vi "PID+calculation.vi"() -> ()   [LabVIEW 2020]
uses:
  Control 1.ctl
  <vilib>/Instr/_visa.llb/VISA Configure Serial Port (Instr).vi
panel:
  in  "Accept":bool
  out "Autotuned":T1
  out "T":dbl=50.98039215686275
  out "L":dbl
  out "Autotune\narray":dbl[](array[numeric])
  in  "Autotune":bool
  out "dt":dbl
  out "String":string
  out "error":dbl=19.0
  out "Error":bool
  out "Numeric":i32=4582
  out "result":dbl(knob)=1.1028626441956932 scale=0.0..255.0
  out "lasterror":dbl=0.010000000000001563
  out "cumError":dbl=0.001016087532043616
  out "previous time":timestamp=timestamp(3700781718.785231 s since 1904-01-01)
  in  "PID Gains":T1={"Proportional Gain(Kp)"=80.0, "Integral Gain(Ki)"=100.0, "Differential Gain(Kd)"=0.0} {"Differential Gain(Kd)" format="%#.6g"; "Integral Gain(Ki)" format="%#.6g"; "Proportional Gain(Kp)" format="%#.6g"}
  in  "VISA resource":refnum<visa-resource-name>="COM11"
  out "PV":dbl(slide)=31.99 scale=0.0..200.0
  in  "SP":T2=32.0 min=0.0 max=0.0 scale=0.0..200.0
  out "SP and PV":cluster{"initial PV":dbl, "SP1:":dbl}(graph)={"initial PV"=31.99, "SP1:"=32.0}
  out "before \ntemp":string="31.99"
  out "remain\nvalue":string
  in  "stop":bool
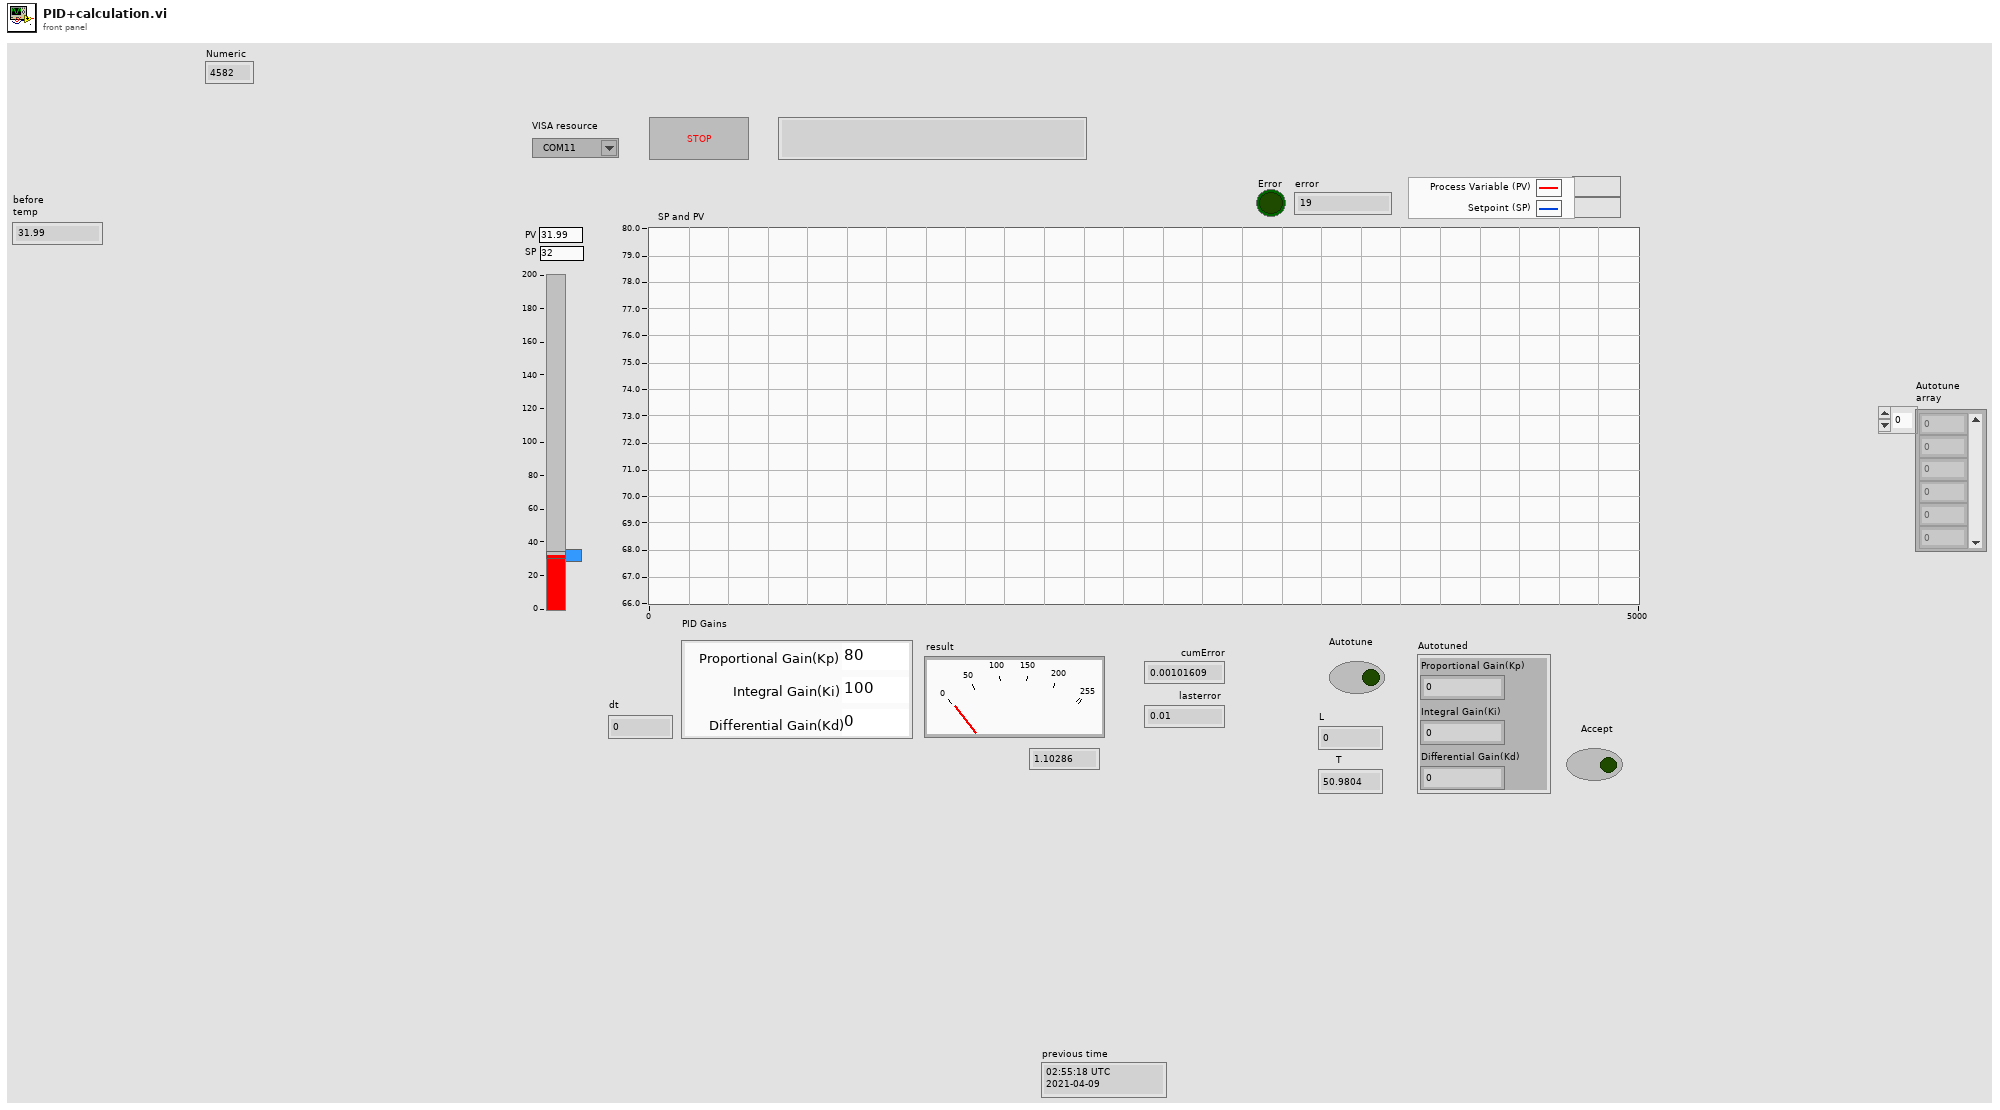
[diagram p1: front panel]
types:
  T1 = cluster{"Proportional Gain(Kp)":dbl, "Integral Gain(Ki)":dbl, "Differential Gain(Kd)":dbl}
  T2 = typedef "Control 1.ctl" = dbl
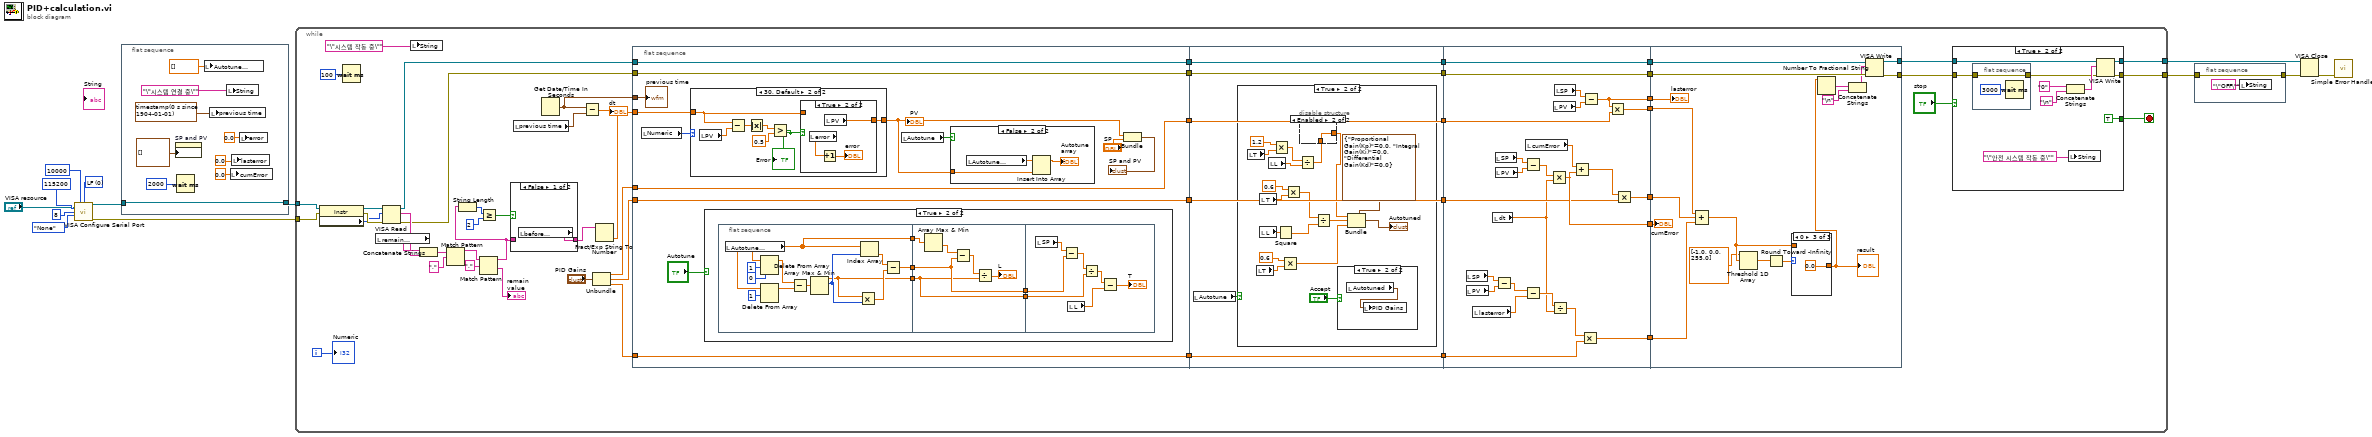
[diagram p0: block diagram]
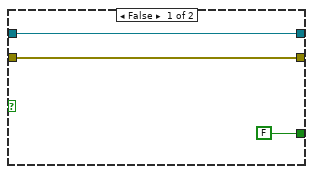
[diagram p2: hidden frame]
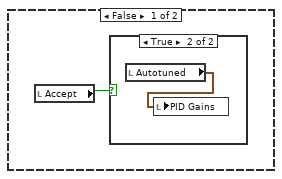
[diagram p7: hidden frame]
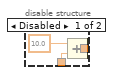
[diagram p10: hidden frame]
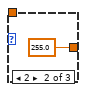
[diagram p12: hidden frame]
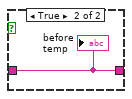
[diagram p13: hidden frame]
diagram:
  w11 = u16 0 items=["LF"]
  n1 = call-poly "VISA Configure Serial Port"("VISA resource name"="VISA resource", "timeout (10sec)"=u32 10000, "termination char\n(0xA = '\\n' = LF)"=w11, "baud rate (9600)"=u32 115200, "data bits (8)"=u16 8, "parity (0:none)"=enum16{"None", "Odd", "Even", "Mark", "Space"}."None") -> ("VISA resource name out"=w13:refnum<visa-resource-name>, "error out"=w4:errorcluster)  [unwired: 8 in]
  n2 = flat-sequence {
    tunnel: w13 -> [w21]
    tunnel: [w21] -> w5
    frame #0 {
      n3 = property on="SP and PV" class="WFChart (strict)"("History Data"=cluster{"initial PV":dbl, "SP1:":dbl}[] []) -> ()  [unwired: 2 in, 2 out]
      n4 = Wait (ms)(milliseconds to wait=u32 2000 ("대기 시간(ms)")) -> ()  [unwired: 1 out]
      n5 = local write "Autotune\narray"(dbl[] [] ("Autotune\narray")) -> ()
      n6 = local write "previous time"(timestamp(0 s since 1904-01-01) ("previous time")) -> ()
      n7 = local write "String"("\"시스템 연결 중\"") -> ()
      n8 = local write "cumError"(0.0 ("cumError")) -> ()
      n9 = local write "lasterror"(0.0 ("lasterror")) -> ()
      n10 = local write "error"(0.0 ("error")) -> ()
    }
  }
  n11 = while {
    tunnel: w5 -> [w59]
    tunnel: w4 -> [w58]
    tunnel: [w38] -> w3
    tunnel: [w37] -> w1
    i -> [w44]
    stop <- w41 stop-if-true
    n12 = property class="Instr"(reference=w59, error in=w58) -> (reference out=w74:refnum<visa-resource-name>, error out=w73:errorcluster, "Serial Settings:Number of Bytes at Serial Port"=w72:u32)
    n13 = Wait (ms)(milliseconds to wait=u32 100 ("대기 시간(ms)")) -> ()  [unwired: 1 out]
    n14 = local read "remain\nvalue"() -> (w71:string)
    n15 = VISA Read(VISA resource name=w74, byte count=w72, error in (no error)=w73) -> (VISA resource name out=w49:refnum<visa-resource-name>, read buffer=w67:string, error out=w46:errorcluster)  [unwired: 1 out]
    n16 = local write "String"("\"시스템 작동 중\"") -> ()
    n17 = Concatenate Strings(w71, w67) -> (w68:string)
    n18 = Match Pattern(string=w68, regular expression=",") -> (before substring=w61:string)  [unwired: 1 in, 3 out]
    n19 = Match Pattern(string=w61, regular expression=",") -> (before substring=w63:string, after substring=→"remain\nvalue":string)  [unwired: 1 in, 2 out]
    n20 = String Length(string=w63) -> (length=w65:i32)
    n21 = Greater Or Equal?(x=w65, y=2) -> (x >= y?=w62:bool)
    n22 = case shown="False" w62 {
      tunnel: [w224 w225] -> w43
      tunnel: w63 -> [_ w225]
      frame False {
        n23 = local read "before \ntemp"() -> (w224:string)
      }
      frame True {
        "before \ntemp" <- w225
      }
    }
    n24 = local read "previous time"() -> (w25:timestamp)
    n25 = Get Date/Time In Seconds() -> (seconds since 1Jan1904=w23:timestamp)
    n26 = Subtract(x=w23, y=w25) -> (x-y=→"dt":dbl)
    n27 = Unbundle("PID Gains") -> ("Proportional Gain(Kp)"=w57:dbl, "Integral Gain(Ki)"=w56:dbl, "Differential Gain(Kd)"=w55:dbl)
    n28 = Fract/Exp String To Number(string=w43) -> (number=w45:dbl)  [unwired: 3 in, 1 out]
    n29 = flat-sequence {
      tunnel: w46 -> [w98]
      tunnel: w49 -> [w99]
      tunnel: w45 -> [w100]
      tunnel: w55 -> [w101]
      tunnel: w56 -> [w102]
      tunnel: w57 -> [w103]
      tunnel: [w103] -> w35
      tunnel: [w102] -> w33
      tunnel: [w101] -> w31
      tunnel: [w99] -> w29
      tunnel: [w98] -> w27
      tunnel: w23 -> [w94]
      tunnel: w35 -> [w154]
      tunnel: [w154] -> w34
      tunnel: w33 -> [w153]
      tunnel: [w153] -> w32
      tunnel: w31 -> [w152]
      tunnel: [w152] -> w30
      tunnel: w29 -> [w151]
      tunnel: [w151] -> w28
      tunnel: w27 -> [w150]
      tunnel: [w150] -> w26
      tunnel: [w197] -> w54
      tunnel: [w193] -> w53
      tunnel: [w185] -> w52
      tunnel: [w184] -> w51
      tunnel: [w183] -> w50
      tunnel: [w182] -> w48
      tunnel: [w181] -> w47
      tunnel: w34 -> [w201]
      tunnel: w32 -> [w194]
      tunnel: w30 -> [w186]
      tunnel: w28 -> [w182]
      tunnel: w26 -> [w181]
      tunnel: w54 -> [w220]
      tunnel: w53 -> [w219]
      tunnel: w52 -> [w218]
      tunnel: w51 -> [w217]
      tunnel: w50 -> [w216]
      tunnel: [w213] -> w40
      tunnel: w48 -> [w215]
      tunnel: [w212] -> w39
      tunnel: w47 -> [w214]
      frame #0 {
        n30 = local read "Numeric"() -> (w95:i32)
        n31 = case shown="30, Default" w95 {
          tunnel: [w137 w140] -> w93
          tunnel: w100 -> [w137 w139]
          frame 0..29 {
          }
          frame 30, Default {
            n32 = local read "PV"() -> (w144:dbl)
            n33 = Subtract(x=w139, y=w144) -> (x-y=w143:dbl)
            n34 = Absolute Value(x=w143) -> (abs(x)=w142:dbl)
            n35 = Greater?(x=w142, y=0.5) -> (0:w138:bool)
            "Error" <- w138
            n36 = case shown="True" w138 {
              tunnel: [w145 w147] -> w140
              tunnel: w139 -> [w145 _]
              frame False {
              }
              frame True {
                n37 = local read "error"() -> (w146:dbl)
                n38 = Increment(x=w146) -> (x+1=→"error":dbl)
                n39 = local read "PV"() -> (w147:dbl)
              }
            }
          }
        }
        "PV" <- w93
        n40 = case shown="True" "Autotune" {
          frame False {
          }
          frame True {
            n41 = flat-sequence {
              tunnel: [w114] -> w111
              tunnel: [w113] -> w110
              tunnel: [w112] -> w109
              tunnel: w111 -> [w125]
              tunnel: w110 -> [w127]
              tunnel: w109 -> [w126]
              tunnel: [w127] -> w108
              tunnel: [w126] -> w107
              tunnel: w108 -> [w135]
              tunnel: w107 -> [w133]
              frame #0 {
                n42 = local read "Autotune\narray"() -> (w114:dbl[])
                n43 = Delete From Array(array=w114, length=1, index=0) -> (array with subset deleted=w121:dbl[])  [unwired: 1 out]
                n44 = Delete From Array(array=w114, length=1) -> (array with subset deleted=w120:dbl[])  [unwired: 1 in, 1 out]
                n45 = Subtract(x=w121, y=w120) -> (x-y=w118:dbl[])
                n46 = Array Max & Min(array=w118) -> (max value=w112:dbl, max index (indices)=w117:i32)  [unwired: 2 out]
                n47 = Multiply(x=w112, y=w117) -> (x*y=w115:dbl)
                n48 = Index Array(array=w114, index=w117) -> (element=w116:dbl)
                n49 = Subtract(x=w116, y=w115) -> (x-y=w113:dbl)
              }
              frame #1 {
                n50 = Array Max & Min(array=w125) -> (min value=w124:dbl)  [unwired: 3 out]
                n51 = Subtract(x=w124, y=w127) -> (x-y=w129:dbl)
                n52 = Divide(x=w129, y=w126) -> (x/y=→"L":dbl)
              }
              frame #2 {
                n53 = local read "SP"() -> (w136:T2)
                n54 = Subtract(x=w136, y=w135) -> (x-y=w134:T2)
                n55 = local read "L"() -> (w131:dbl)
                n56 = Divide(x=w134, y=w133) -> (x/y=w132:T2)
                n57 = Subtract(x=w132, y=w131) -> (x-y=→"T":T2)
              }
            }
          }
        }
        n58 = local read "Autotune"() -> (w91:bool)
        n59 = case shown="False" w91 {
          tunnel: w93 -> [_ w106]
          frame True {
          }
          frame False {
            n60 = local read "Autotune\narray"() -> (w104:dbl[])
            n61 = Insert Into Array(array=w104, new element=w106) -> (→"Autotune\narray":dbl[])  [unwired: 1 in]
          }
        }
        n62 = Bundle("PV"=w93, "SP"="SP") -> (→"SP and PV":cluster{"PV":dbl, "SP":T2})  [unwired: 1 in]
        "previous time" <- w94
      }
      frame #1 {
        n63 = local read "Autotune"() -> (w149:bool)
        n64 = case shown="True" w149 {
          frame False {
            n65 = local read "Accept"() -> (w155:bool)
            n66 = case shown="True" w155 {
              frame False {
              }
              frame True {
                n67 = local read "Autotuned"() -> (w156:T1)
                n68 = local write "PID Gains"(w156) -> ()
              }
            }
          }
          frame True {
            n69 = local read "T"() -> (w174:dbl)
            n70 = local read "T"() -> (w167:dbl)
            n71 = local read "T"() -> (w166:dbl)
            n72 = local read "L"() -> (w168:dbl)
            n73 = local read "L"() -> (w171:dbl)
            n74 = Multiply(x=1.2, y=w174) -> (x*y=w172:dbl)
            n75 = Square(x=w168) -> (x^2=w163:dbl)
            n76 = Multiply(x=0.6, y=w167) -> (x*y=w169:dbl)
            n77 = Multiply(x=0.6, y=w166) -> (x*y=w164:dbl)
            n78 = Divide(x=w172, y=w171) -> (x/y=w158:dbl)
            n79 = disable-structure shown="Enabled" {
              disable-tunnel: [w178 w179] -> w159
              disable-tunnel: w158 -> [w177 w179]
              frame Disabled {
                n80 = Add(x=10.0, y=w177) -> (x+y=w178:dbl)
              }
              frame Enabled {
              }
            }
            n81 = Divide(x=w164, y=w163) -> (x/y=w162:dbl)
            n82 = case shown="True" "Accept" {
              frame False {
              }
              frame True {
                n83 = local read "Autotuned"() -> (w175:T1)
                n84 = local write "PID Gains"(w175) -> ()
              }
            }
            n85 = Bundle(cluster=T1 {"Proportional Gain(Kp)"=0.0, "Integral Gain(Ki)"=0.0, "Differential Gain(Kd)"=0.0} ("PID gains"), "Proportional Gain(Kp)"=w159, "Integral Gain(Ki)"=w162, "Differential Gain(Kd)"=w169) -> (→"Autotuned":T1)
          }
        }
      }
      frame #2 {
        n86 = local read "SP"() -> (w192:T2)
        n87 = local read "PV"() -> (w191:dbl)
        n88 = local read "lasterror"() -> (w189:dbl)
        n89 = local read "dt"() -> (w180:dbl)
        n90 = local read "SP"() -> (w200:T2)
        n91 = local read "PV"() -> (w199:dbl)
        n92 = Subtract(x=w192, y=w191) -> (x-y=w190:T2)
        n93 = Subtract(x=w200, y=w199) -> (x-y=w198:T2)
        n94 = Subtract(x=w190, y=w189) -> (x-y=w188:T2)
        n95 = local read "cumError"() -> (w196:dbl)
        n96 = Multiply(x=w198, y=w180) -> (x*y=w197:T2)
        n97 = Divide(x=w188, y=w180) -> (x/y=w187:T2)
        n98 = local read "PV"() -> (w203:dbl)
        n99 = local read "SP"() -> (w202:T2)
        n100 = Add(x=w196, y=w197) -> (x+y=w195:T2)
        n101 = Multiply(x=w187, y=w186) -> (x*y=w183:T2)
        n102 = Subtract(x=w202, y=w203) -> (x-y=w193:T2)
        n103 = Multiply(x=w193, y=w201) -> (x*y=w185:T2)
        n104 = Multiply(x=w195, y=w194) -> (x*y=w184:T2)
      }
      frame #3 {
        n105 = Compound Arithmetic op=ADD(w218, w217, w216) -> (w208:T2)
        n106 = Threshold 1D Array(2:w208, 3:dbl[] [-1.0, 0.0, 255.0] ("array of numbers or points")) -> (0:w207:dbl)  [unwired: 1 in]
        n107 = Round Toward -Infinity(1:w207) -> (0:w206:dbl)
        n108 = case shown="0" w206 {
          tunnel: [w221 T2 255.0 ("SP") 0.0 ("result")] -> w205
          tunnel: w208 -> [w221 _ _]
          frame 1, Default {
          }
          frame 2 {
          }
          frame 0 {
          }
        }
        "result" <- w205
        n109 = Number To Fractional String(number=w205) -> (F-format string=w211:string)  [unwired: 3 in]
        n110 = Concatenate Strings(w211, "\n") -> (w209:string)
        n111 = VISA Write(VISA resource name=w215, write buffer=w209, error in (no error)=w214) -> (VISA resource name out=w213:refnum<visa-resource-name>, error out=w212:errorcluster)  [unwired: 1 out]
        "cumError" <- w220
        "lasterror" <- w219
      }
    }
    n112 = case shown="True" "stop" {
      tunnel: [FALSE TRUE] -> w41
      tunnel: [w77 w83] -> w38
      tunnel: w40 -> [w77 w84]
      tunnel: w39 -> [w76 w80]
      tunnel: [w76 w81] -> w37
      frame False {
      }
      frame True {
        n113 = flat-sequence {
          tunnel: [w89] -> w79
          tunnel: w80 -> [w89]
          frame #0 {
            n114 = Wait (ms)(milliseconds to wait=u32 3000) -> ()  [unwired: 1 out]
          }
        }
        n115 = Concatenate Strings("0" ("string"), "\n") -> (w88:string)
        n116 = local write "String"("\"안전 시스템 작동 중\"") -> ()
        n117 = VISA Write(VISA resource name=w84, write buffer=w88, error in (no error)=w79) -> (VISA resource name out=w83:refnum<visa-resource-name>, error out=w81:errorcluster)  [unwired: 1 out]
      }
    }
    "Numeric" <- w44
  }
  n118 = flat-sequence {
    tunnel: [w226] -> w2
    tunnel: w1 -> [w226]
    frame #0 {
      n119 = local write "String"("\"OFF\"") -> ()
    }
  }
  n120 = VISA Close(VISA resource name=w3, error in (no error)=w2) -> (error out=w7:errorcluster)
  n121 = call <vilib>:"Simple Error Handler.vi"("error in (no error)"=w7) -> ()  [unwired: 4 in, 5 out]
